vi "(SubVI) Set Scanrate and Pull_PI_YCC.vi"(0 "toward+ ?\nT=+, F=-":bool, 2 "axis":u32=1, 3 "scan rate  (um/s)":dbl=2.0 format="%.3f", 5 "range  (um)":dbl=2.0 min=0.0 max=100.0 step=0.5 format="%.3f") -> (6 "Start From  (um)":dbl min=0.0 max=100.0 step=0.5 format="%.3f", 7 "Traveling time (s)":dbl)   [LabVIEW 2014]
panel:
  out "Velocity":dbl[](array[numeric]) format="%.6f"
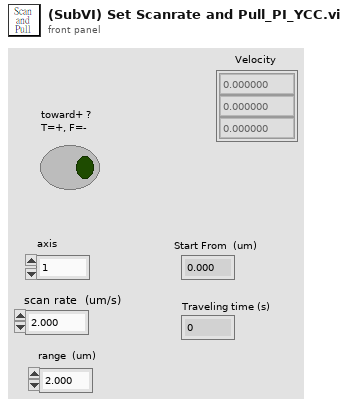
[diagram p1: front panel]
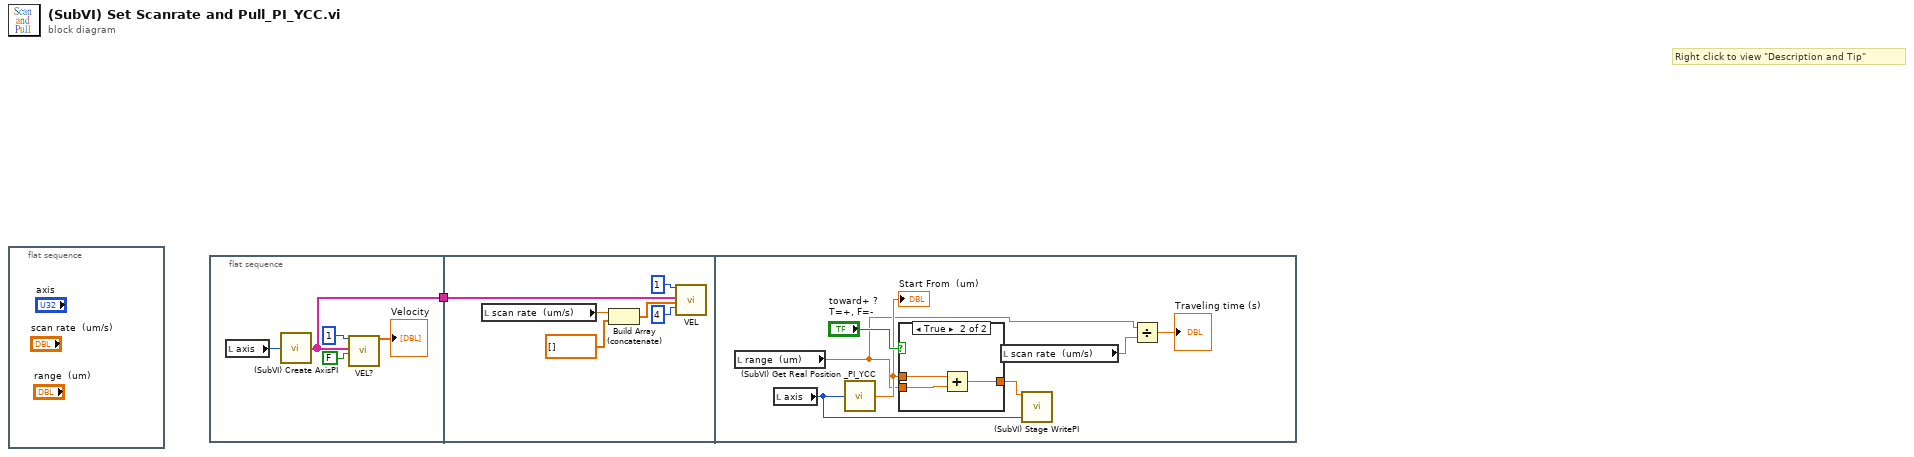
[diagram p0: block diagram]
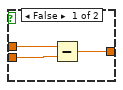
[diagram p2: hidden frame]
diagram:
  # "Right click to view \"Description and Tip\""
  n1 = flat-sequence {
    frame #0 {
    }
  }
  n2 = flat-sequence {
    tunnel: [w3] -> w1
    tunnel: w1 -> [w7]
    frame #0 {
      n3 = local read "axis"() -> (w2:u32)
      n4 = call "(SubVI) Create AxisPI.vi"("axis"=w2) -> ("Axis String Array"=w3:string[])  [unwired: 2 in, 2 out]
      n5 = call "VEL?.vi"("System no."=1, "Axes to query"=w3, "All axes?"=FALSE) -> ("Velocity"=→"Velocity":dbl[])  [unwired: 15 in, 1 out]
    }
    frame #1 {
      n6 = local read "scan rate  (um/s)"() -> (w8:dbl)
      n7 = Build Array (concatenate)(w8, dbl[] []) -> (w10:dbl[])
      n8 = call "VEL.vi"("System no."=1, "Axes to set"=w7, "Velocity values"=w10, "No.of digits"=i16 4) -> ()  [unwired: 14 in, 2 out]
    }
    frame #2 {
      n9 = local read "range  (um)"() -> (w15:dbl)
      n10 = local read "axis"() -> (w17:u32)
      n11 = call "(SubVI) Get Real Position _PI_YCC.vi"("Axis"=w17) -> ("Real Current Commanded position (um)"=w16:dbl)  [unwired: 4 in]
      "Start From  (um)" <- w16
      n12 = case shown="True" "toward+ ?\nT=+, F=-" {
        tunnel: w16 -> [w22 w25]
        tunnel: [w21 w24] -> w18
        tunnel: w15 -> [w20 w23]
        frame False {
          n13 = Subtract(x=w22, y=w20) -> (x-y=w21:dbl)
        }
        frame True {
          n14 = Add(x=w25, y=w23) -> (x+y=w24:dbl)
        }
      }
      n15 = local read "scan rate  (um/s)"() -> (w14:dbl)
      n16 = call "(SubVI) Stage WritePI.vi"("axis"=w17, "position"=w18) -> ()  [unwired: 4 in]
      n17 = Divide(x=w15, y=w14) -> (x/y=→"Traveling time (s)":dbl)
    }
  }
